vi "Is Negative Infinity.vi"(1 "Numeric":dbl) -> (0 "is minus infinity":bool)   [LabVIEW 2015]
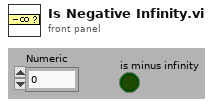
[diagram p1: front panel]
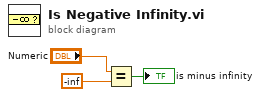
[diagram p0: block diagram]
diagram:
  n1 = Equal?(x="Numeric", y=-inf) -> (x = y?=→"is minus infinity":bool)
